vi "Set U64 Package Attribute Value.vi"(6 "add nonexisting attribute to string (T)":bool=TRUE, 8 "error in (no error)":errorcluster, 9 "package attribute value":u64, 10 "package attribute name":string, 11 "package attributes string in":string) -> (0 "error out":errorcluster, 1 "attribute found?":bool, 2 "new attribute added to string?":bool, 3 "package attributes string out":string)   [LabVIEW 2014, in "NIPM_API.lvlib"]
doc: "Sets the value for an attribute in a package attribute string.\n\npackage attributes string in - This is the initial string containing the package attributes. For example, this string could come from reading the contents of an unpacked package's control file.\n\npackage attribute name - This is the name of the attribute whose value you want to change.\n\npackage attribute value - This is the value you want to set the attribute to.\n\nadd nonexisting attribute to string - If this VI does not find the \"package attribute name\" in the \"package attributes string in\" string, this input determines whether this VI will add the \"package attribute name\" and \"package attribute value\" to the \"package attribute string\".\nNote: If this input is TRUE, but the \"package attribute value\" is a default value (0), then this VI will not add a new attribute to the string.\n\nnew attribute added to string? - This output will be TRUE if a new attribute (did not exist in the incoming \"package attributes string in\" string) was added to the package attributes string.\n\nattribute found? - This output will be TRUE if the \"package attribute name\" was found in the incoming \"package attributes string in\" string."
uses:
  NIPM_API.lvlib
  <vilib>/Utility/error.llb/whitespace.ctl
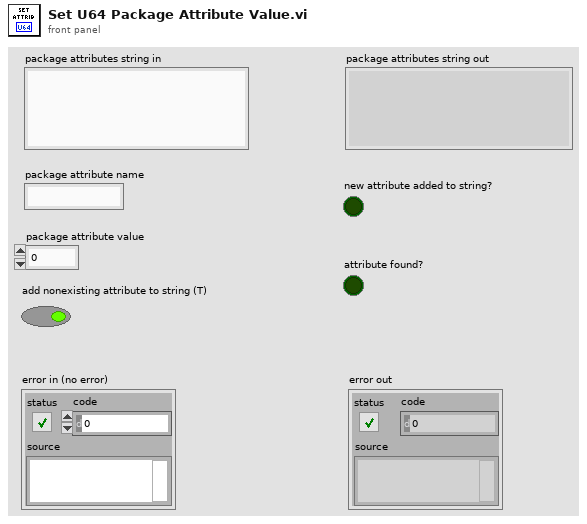
[diagram p1: front panel]
types:
  T1 = typedef "whitespace.ctl" = u16
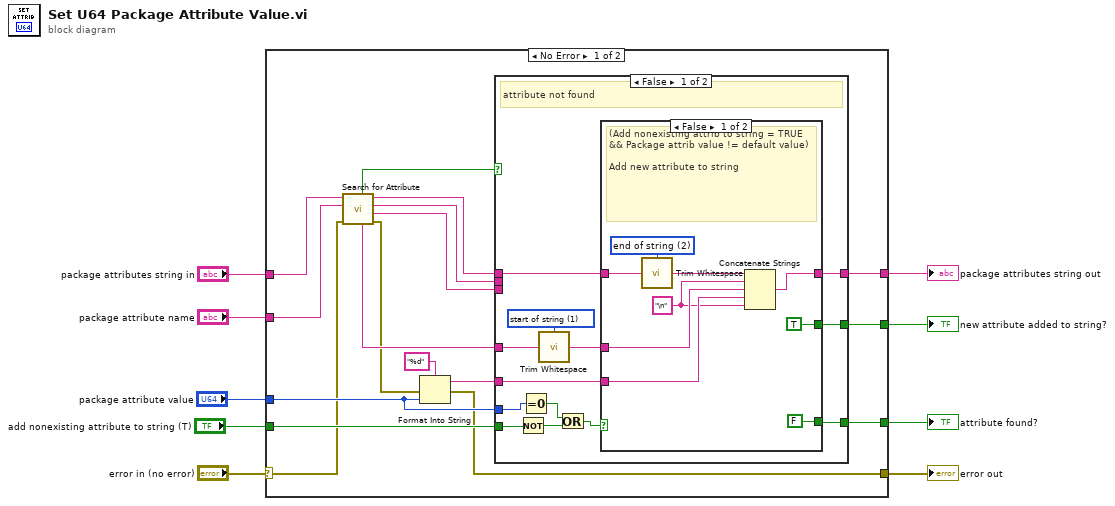
[diagram p0: block diagram]
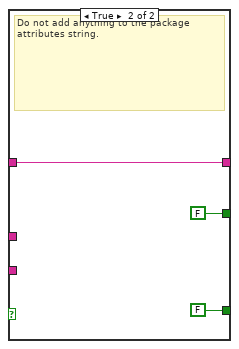
[diagram p2: hidden frame]
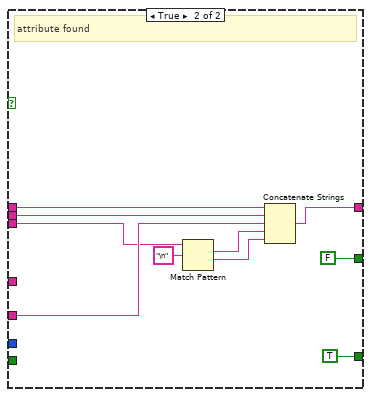
[diagram p3: hidden frame]
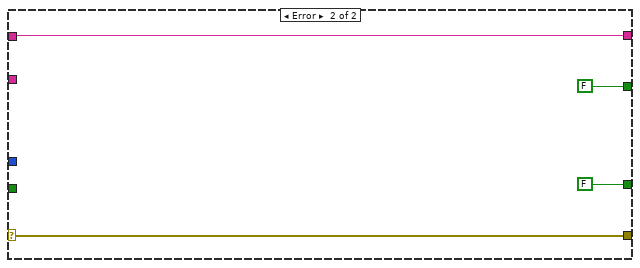
[diagram p4: hidden frame]
diagram:
  n1 = case shown="No Error" "error in (no error)" {
    selector: "error in (no error)" -> [w11 w65]
    tunnel: [w26 w62] -> w4
    tunnel: "package attribute name" -> [w13 _]
    tunnel: "package attributes string in" -> [w15 w62]
    tunnel: [w10 w65] -> w1
    tunnel: "package attribute value" -> [w20 _]
    tunnel: [w25 FALSE] -> w6
    tunnel: "add nonexisting attribute to string (T)" -> [w24 _]
    tunnel: [w23 FALSE] -> w5
    frame No Error {
      n2 = call "Search for Attribute.vi"("error in (no error)"=w11, "package attribute name"=w13, "package attributes CLI string in"=w15) -> ("error out"=w12:errorcluster, "string after attribute"=w16:string, "string matching attribute"=w17:string, "string before attribute"=w18:string, "package attribute string"=w14:string, "attribute found?"=w19:bool)  [unwired: 3 in]
      n3 = Format Into String(format string="%d", error in=w12, w20) -> (resulting string=w22:string, error out=w10:errorcluster)  [unwired: 1 in]
      n4 = case shown="False" w19 {
        tunnel: w18 -> [w39 w61]
        tunnel: w17 -> [_ w60]
        tunnel: w22 -> [w35 w59]
        tunnel: w16 -> [_ w58]
        tunnel: [w37 w56] -> w26
        tunnel: [w38 FALSE] -> w25
        tunnel: w14 -> [w36 _]
        tunnel: w24 -> [w32 _]
        tunnel: [w34 TRUE] -> w23
        tunnel: w20 -> [w29 _]
        frame False {
          w27 = T1 1 items=["both", "start of string", "end of string"] ("location (both)")
          # "attribute not found"
          n5 = Not(x=w32) -> (.not. x?=w33:bool)
          n6 = Equal To 0?(x=w29) -> (x = 0?=w30:bool)
          n7 = call <vilib>:"Trim Whitespace.vi"("string"=w36, "location (both)"=w27) -> ("trimmed string"=w28:string)
          n8 = Or(x=w30, y=w33) -> (x .or. y?=w31:bool)
          n9 = case shown="False" w31 {
            tunnel: w39 -> [w48 w51]
            tunnel: [TRUE FALSE] -> w38
            tunnel: [w46 w51] -> w37
            tunnel: w28 -> [w45 _]
            tunnel: w35 -> [w44 _]
            tunnel: [FALSE FALSE] -> w34
            frame False {
              w41 = "\n"
              w42 = T1 2 items=["both", "start of string", "end of string"] ("location (both)")
              # "(Add nonexisting attrib to string = TRUE && Package attrib value != default value)\n\nAdd new attribute to string"
              n10 = call <vilib>:"Trim Whitespace.vi"("string"=w48, "location (both)"=w42) -> ("trimmed string"=w43:string)
              n11 = Concatenate Strings(w43, w41, w45, w44, w41) -> (w46:string)
            }
            frame True {
              # "Do not add anything to the package attributes string."
            }
          }
        }
        frame True {
          # "attribute found"
          n12 = Match Pattern(string=w58, regular expression="\n") -> (match substring=w54:string, after substring=w53:string)  [unwired: 1 in, 2 out]
          n13 = Concatenate Strings(w61, w60, w59, w54, w53) -> (w56:string)
        }
      }
    }
    frame Error {
    }
  }
  "error out" <- w1
  "package attributes string out" <- w4
  "new attribute added to string?" <- w6
  "attribute found?" <- w5
